vi "OriginalDigitizerLiveNew.vi"() -> ()   [LabVIEW 2020]
doc: "Example Description:\nThis example demonstrates how to enable Time Interleaved Sampling with the NI 5772 adapter module to achieve a sampling rate of 1.6GS/s. This example continuously acquires records of analog input data from the NI 5772 adapter module. It allows you to select an AI channel, trigger type, and record size. This VI must be compiled before it is run. \n\nRunning the VI:\nThis VI must be run from the NI 5772 - Getting Started (Host).vi. Refer to the host VI documentation for steps regarding running and configuring the FPGA VI. \n\nExecution Steps:\nRefer to the Block Diagram of this VI for execution comments."
uses:
  Controls/AI Trigger Type.ctl
  Controls/Aquire State.ctl
  Controls/DigitizerState.ctl
  <vilib>/Platform/TimedLoop/XDataNode/timing_clust.ctl
  <vilib>/Platform/TimedLoop/XDataNode/nitl_modes.ctl
  <vilib>/Platform/TimedLoop/XDataNode/wakeup.ctl
  Controls/NeighbouringAvgStates.ctl
  <vilib>/rvi/Emulation/niFpgaGetClockAttributes.vi
  <vilib>/rvi/Emulation/niFpgaSctlEmulationGetInTimedLoop.vi
  <vilib>/rvi/Emulation/niFpgaEmulationReportErrorSimple.vi
  <vilib>/rvi/eio/common/nirviEmuTemplateMethod_errors.vi
  <vilib>/rvi/Emulation/niFpgaCriticalErrorInLSC.vi
  <vilib>/rvi/Emulation/niFpgaEmulationIsFPGAContextNoSignature.vi
  <vilib>/rvi/errors/niFpgaSetErrorForExecOnDevCompSimple.vi
  <vilib>/rvi/eio/common/nirviEmuReportErrorAndStop.vi
  <vilib>/rvi/DataTransferAndStorage/Container/Common/niFpgaContainerGetUniqueNameForEmu.vi
  <vilib>/rvi/FIFO/Fifo_Resource/nirvififoEmulationSetSize.vi
  <vilib>/rvi/FIFO/Fifo_Resource/nirviFifoEmulationQueueMgr.vi
  <instcachedir>/0/nirviFifoEmulationQueueMgr_E5CAEC123FF24DC58D834DCA3CDAA9B5.lvgen/nirviFifoEmulationQueueMgr_E5CAEC123FF24DC58D834DCA3CDAA9B5_003.vi
  <vilib>/Utility/error.llb/Clear Errors.vi
  <vilib>/rvi/FIFO/Fifo_Resource/nirvififoEmulationCreateLock.vi
  <vilib>/rvi/Emulation/niFpgaProcessEmulError.vi
  <vilib>/rvi/FIFO/Fifo_Resource/nirvififoEmulationObtainLock.vi
  <vilib>/rvi/FIFO/Fifo_Resource/nirvififoEmulationReleaseLock.vi
  <vilib>/rvi/occurrence/nirviWaitOnOccurrenceBase.vi
  <vilib>/rvi/errors/nirviReportUnexpectedCaseInternalError.vi
  <vilib>/rvi/errors/nirviReportUnexpectedCaseInternalError (U32).vi
  <vilib>/rvi/FIFO/Fifo_Resource/nirvififoEmulationDetermineInputValidOut.vi
  <vilib>/rvi/interface/RandomDataEmulation/niFpgaRandomDataHandleErrors.vi
  <instcachedir>/0/nirviFifoEmulationQueueMgr_E5CAEC123FF24DC58D834DCA3CDAA9B5.lvgen/nirviFifoEmulationQueueMgr_E5CAEC123FF24DC58D834DCA3CDAA9B5_004.vi
  <instcachedir>/0/nirviFifoEmulationQueueMgr_E5CAEC123FF24DC58D834DCA3CDAA9B5.lvgen/nirviFifoEmulationQueueMgr_E5CAEC123FF24DC58D834DCA3CDAA9B5_000.vi
  <instrlib>/_niInstr/Basic Elements/v1/FPGA/Private/Count Up U32.vi
  <vilib>/eio/EIONode/EIONode.xnode
  <vilib>/Platform/TimedLoop/XDataNode/XDataNode.xnode
  <vilib>/rvi/DataTransferAndStorage/Container/XNode/niFpgaContainer.xnode
  <vilib>/rvi/FIFO/Fifo_Resource/nirvififoEmulationRead.vi
  <vilib>/rvi/FIFO/Fifo_Resource/nirvififoEmulationWrite.vi
  <vilib>/rvi/interface/RandomDataEmulation/nirviRandomDataFpgaReadWriteTemplate.vi
  <vilib>/Platform/TimedLoop/XDataNode/XDNodeRunTimeDep.lvlib
  <instrlib>/_niInstr/Basic Elements/v1/FPGA/niInstr Basic Elements v1 FPGA.lvlib
panel:
  out "count out":u32
  in  "Trig Width":u32
  in  "vi/nGenTrig":bool
  out "Trig In":u32
  in  "Clear TrigIn Count":bool
  out "Avg State":T1
  out "Element RemovedFIFO":u64
  out "F to H FIFO Overflow? 2":bool caption="FIFO Overflow?"
  in  "Align TimeOut":u16=50
  in  "WaitForWave\nCompletion [cycles]":u16
  out "AvgCount":u16=1
  in  "AvgCount_powerOf2":i16=1
  in  "DS":u8
  in  "Trigger":bool=TRUE
  out "Acquire State":T2
  in  "Delay Cycles":u16=512 caption="Samples Per Trigger" min=1 step=1
  out "TS FIFO In Overflow?":bool caption="FIFO Overflow?"
  in  "Samples Per Trigger":u16=512 min=1 step=1
  in  "Arm Trigger":bool
  in  "User Command Commit":bool
  in  "User Command":u8
  out "User Command Idle":bool
  out "User Command Status":u8
  in  "User Data 0":u16
  in  "User Data 1":u8
  out "PLL Locked":bool
  out "User Error":bool
  out "Configured?":bool
  out "DMA FIFO Overflow?":bool caption="FIFO Overflow?"
  in  "Trigger Level":i16
  in  "Trigger Type":T3
  # "Resource Configuration"
  # "Analog Input"
  # "Clock Configuration"
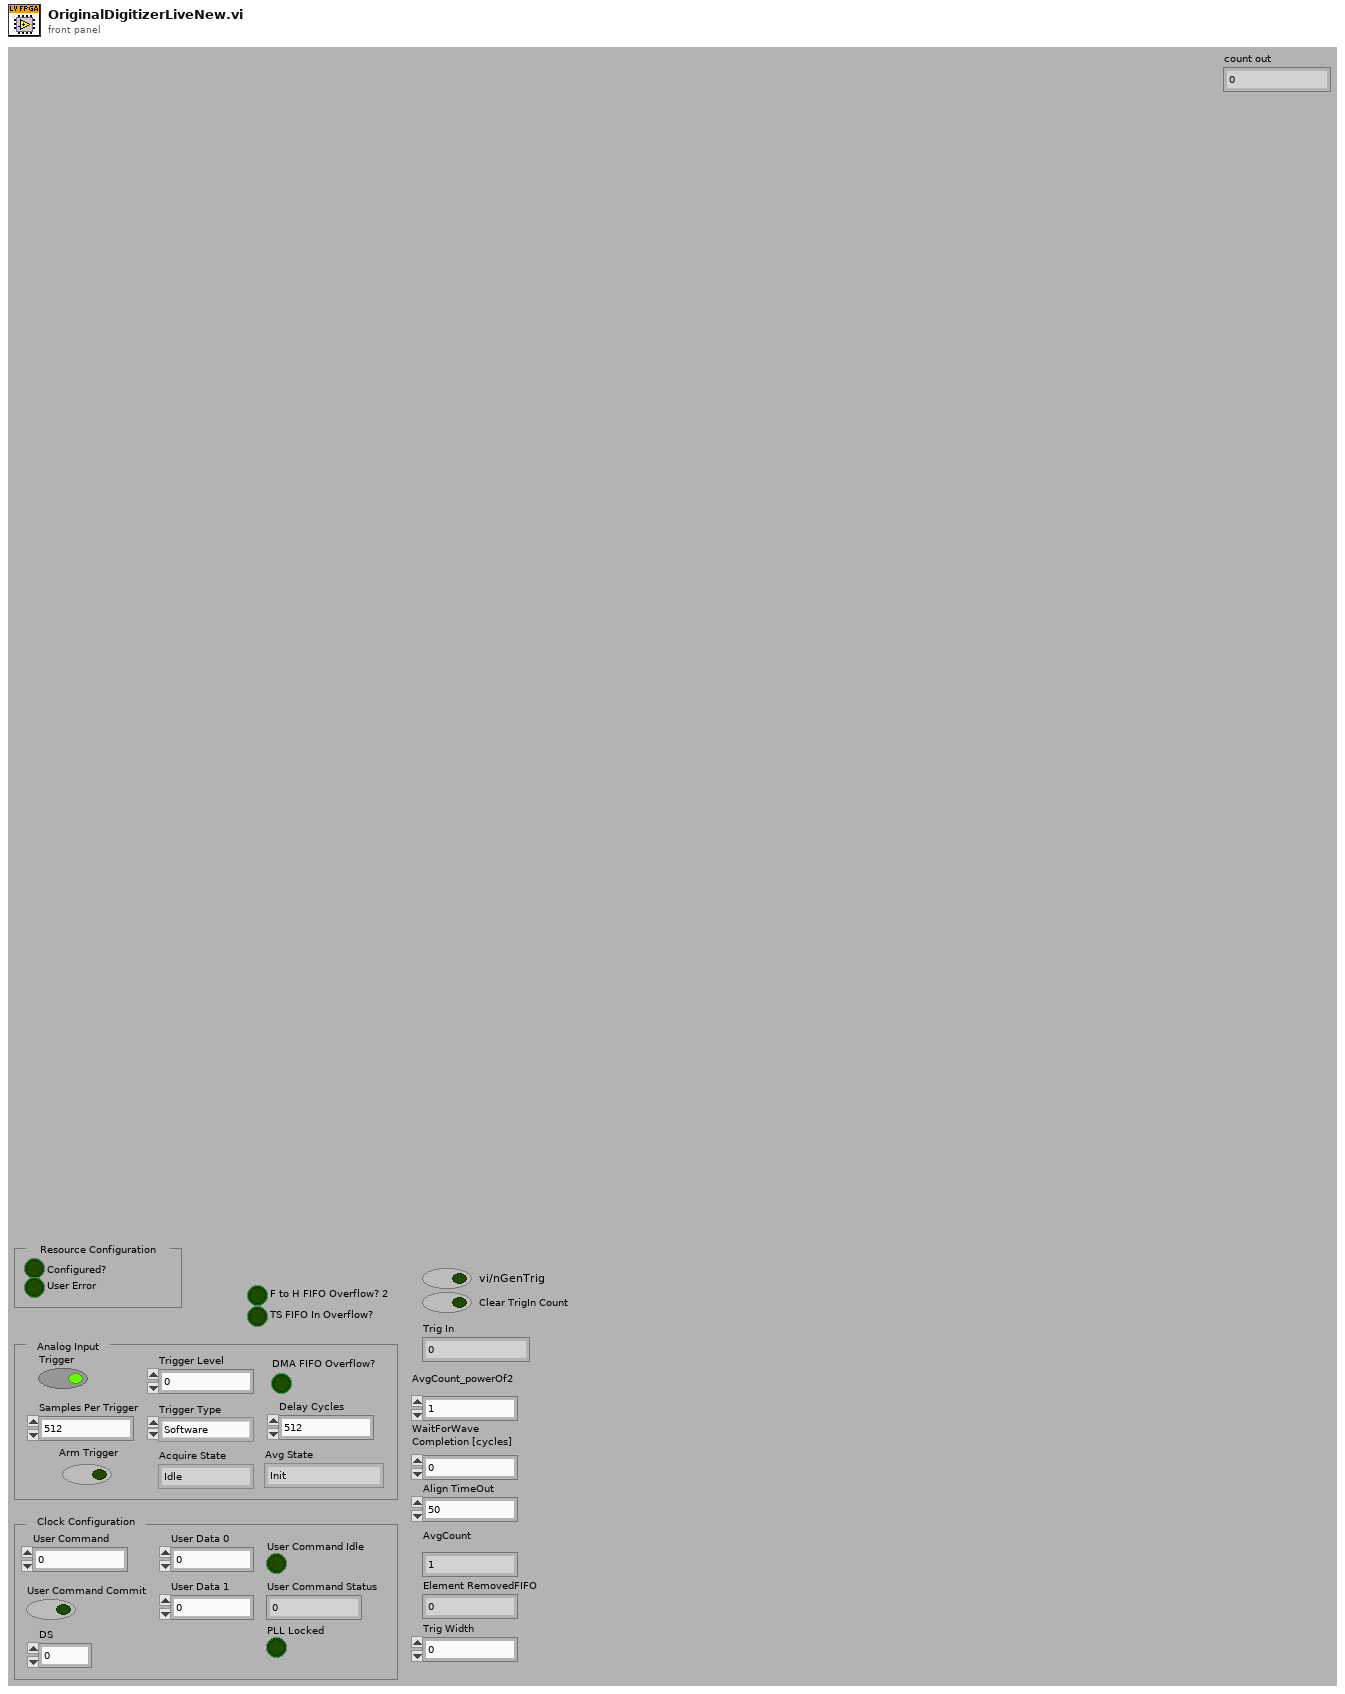
[diagram p1: front panel]
types:
  T1 = typedef "DigitizerState.ctl" = enum16{"Init", "Clear Accumulator", "Build Accumulator", "GetData", "SetData", "AverageCountCheck", "SendtoHost"}
  T2 = typedef "Aquire State.ctl" = enum8{"Idle", "Wait for Trigger", "AlignWave", "Hold Aquire", "Acquire", "WaitForWaveCompletion", "CheckAvg"}
  T3 = typedef "AI Trigger Type.ctl" = enum8{"Software", "Data Edge"}
  T4 = typedef "NeighbouringAvgStates.ctl" = enum16{"Read_noDS", "Write1_noDS", "Write2_noDS"}
  T5 = typedef "XDNodeRunTimeDep.lvlib/timing_clust.ctl" = cluster{"Expected End [f-1]":u64, "Actual End [f-1]":u64, "Finished Late? [f-1]":bool, "Expected End [i-1]":u64, "Actual End [i-1]":u64, "Finished Late? [i-1]":bool, "Expected Start [i]":u64, "Actual Start [i]":u64, "Expected Start [f]":u64, "Actual Start [f]":u64, "Source Name":string, "Structure Name":string, "Period":i64, "Deadline":i64, "Offset":i64, "Start":i64, "Priority":i32, "Timeout":i32, "Mode":T6, "Wakeup Reason":T7, "Error":errorcluster, "Source Type":string, "Secondary Source Type":string, "Global End Time":u64, "Global Start Time":u64, "Frame Duration":u64, "Iteration Duration":u64, "Assigned CPU":i32, "I/O Scan Engine Mode":u32}
  T6 = typedef "XDNodeRunTimeDep.lvlib/nitl_modes.ctl" = enum32{"No Change", "Process missed periods, maintain original phase", "Discard missed periods, maintain original phase", "Process missed periods, ignore original phase", "Discard missed periods, ignore original phase"}
  T7 = typedef "XDNodeRunTimeDep.lvlib/wakeup.ctl" = enum32{"Normal", "Aborted", "Asynchronous wakeup", "Timing source error", "Timed loop error", "Timeout"}
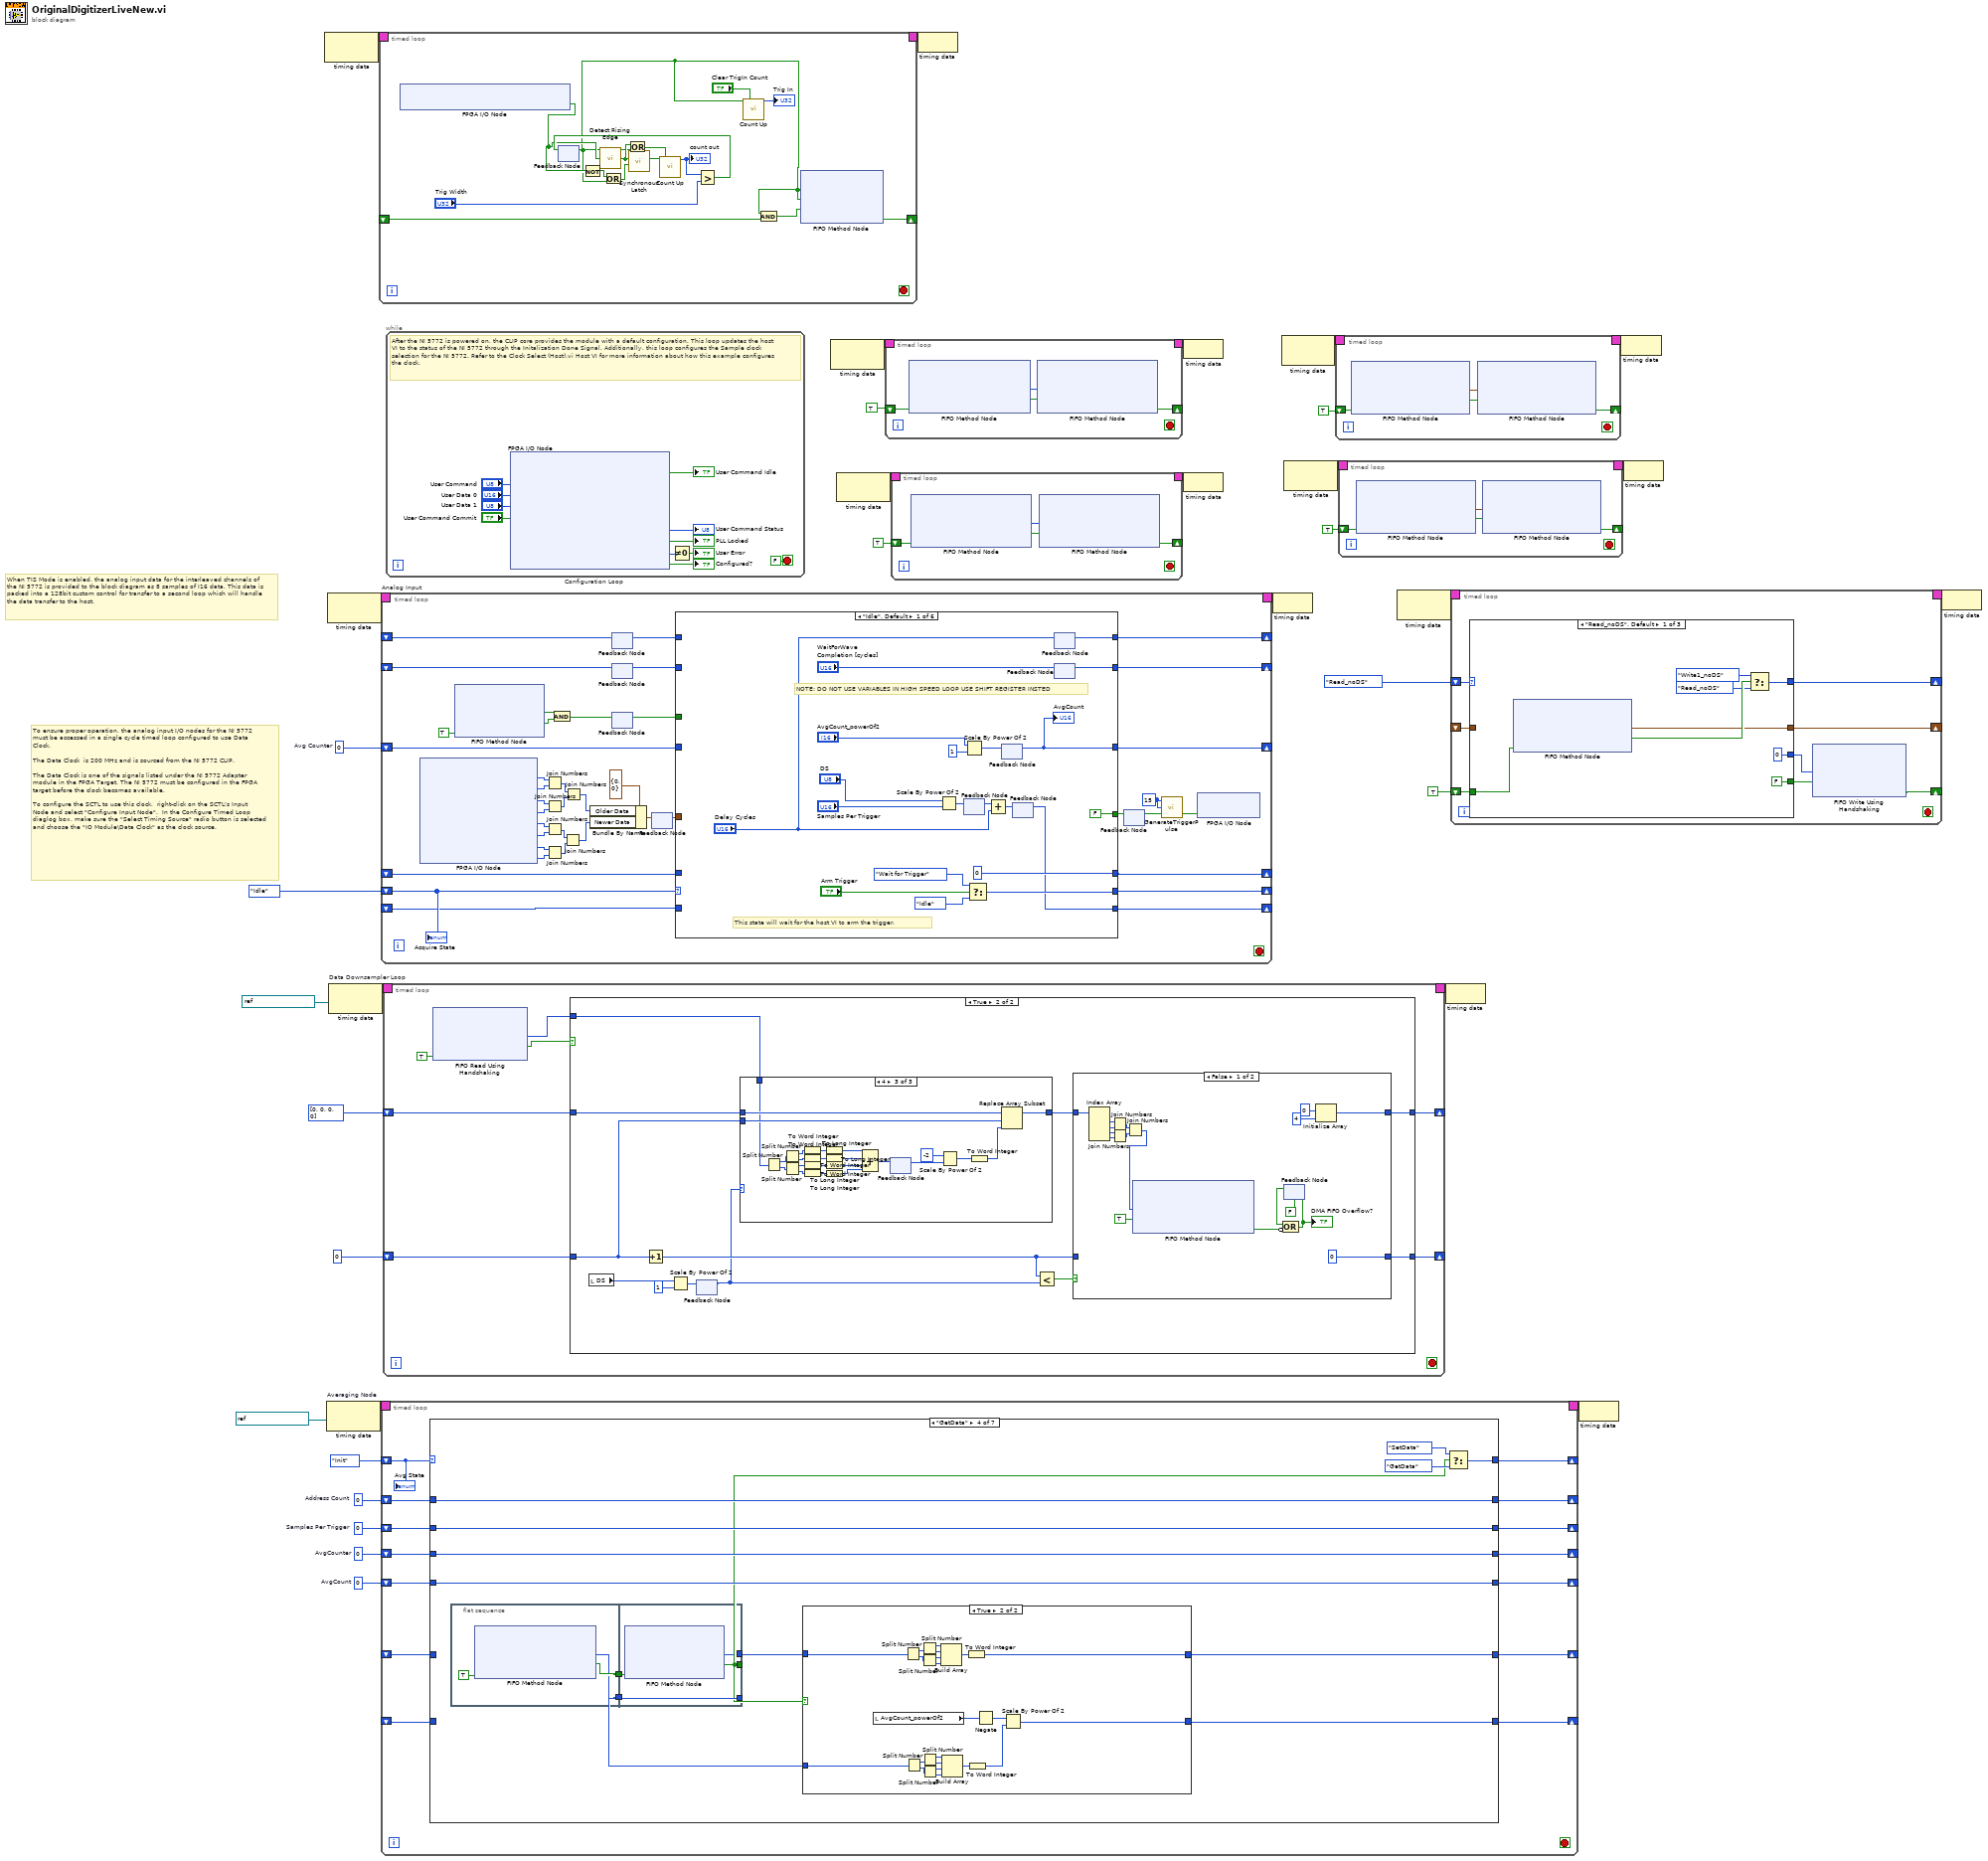
[diagram p0: block diagram]
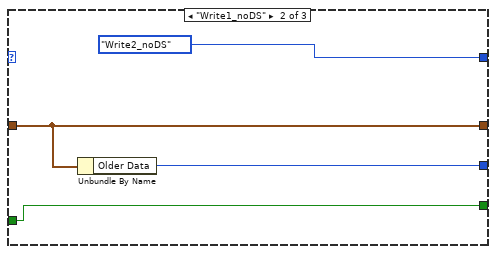
[diagram p2: hidden frame]
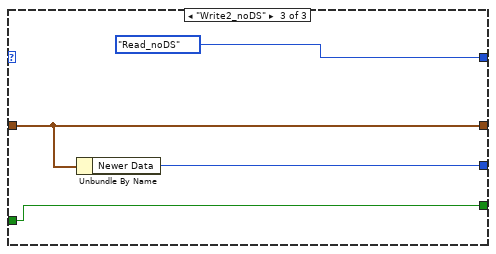
[diagram p3: hidden frame]
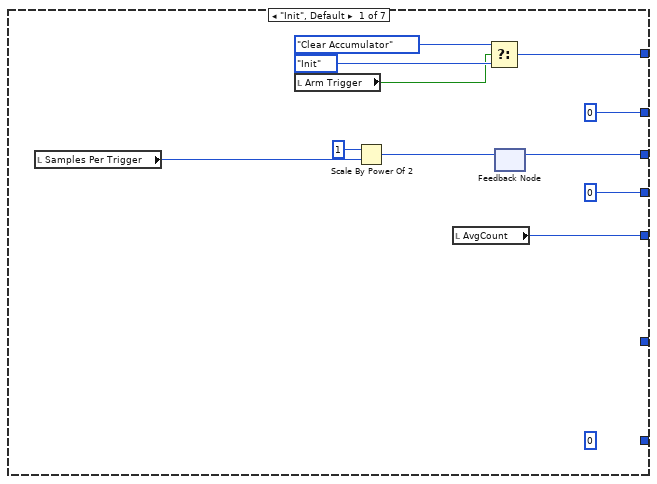
[diagram p4: hidden frame]
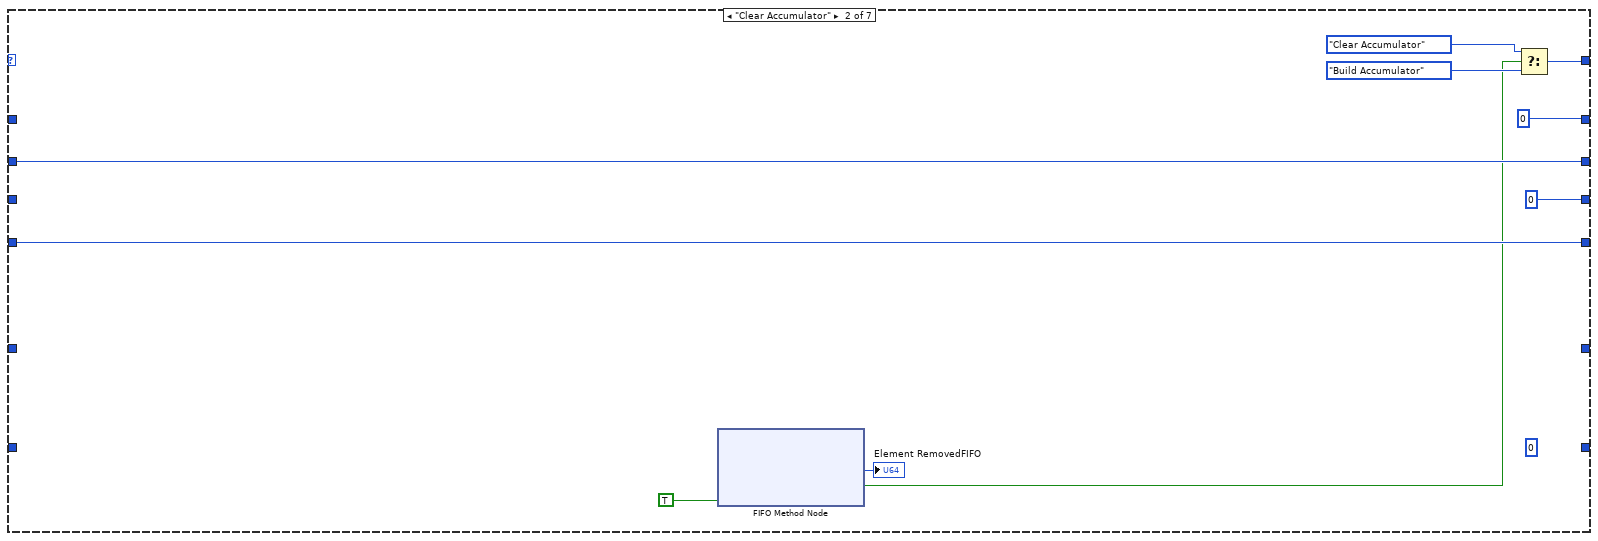
[diagram p5: hidden frame]
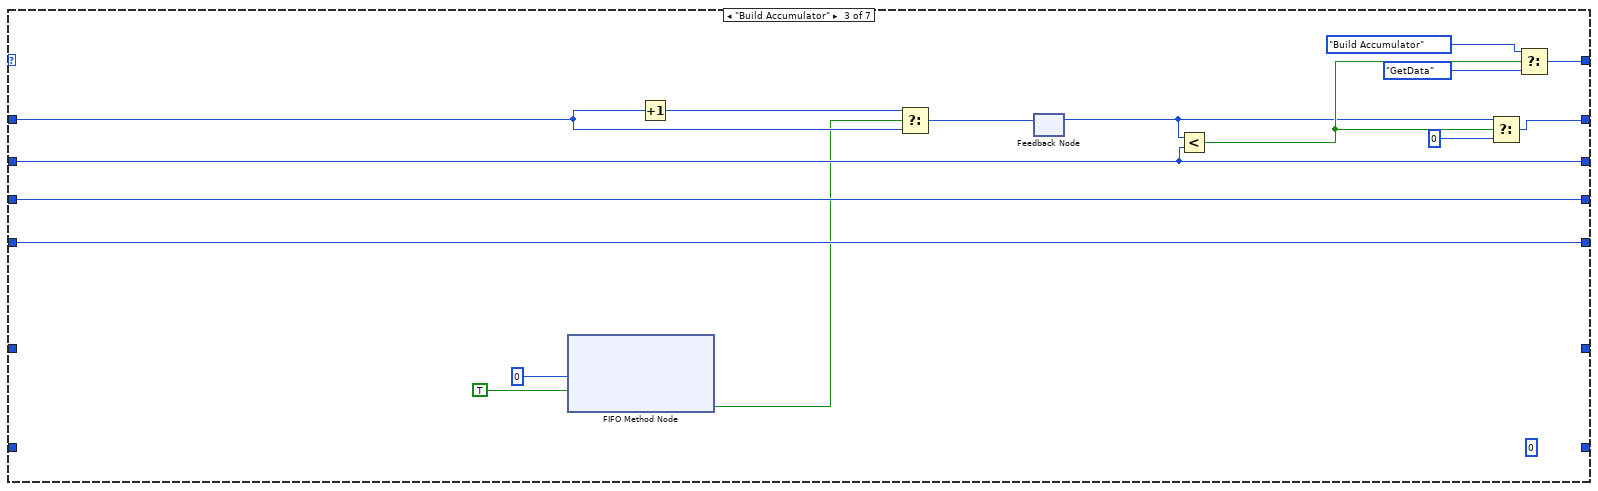
[diagram p6: hidden frame]
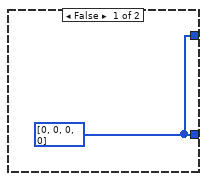
[diagram p7: hidden frame]
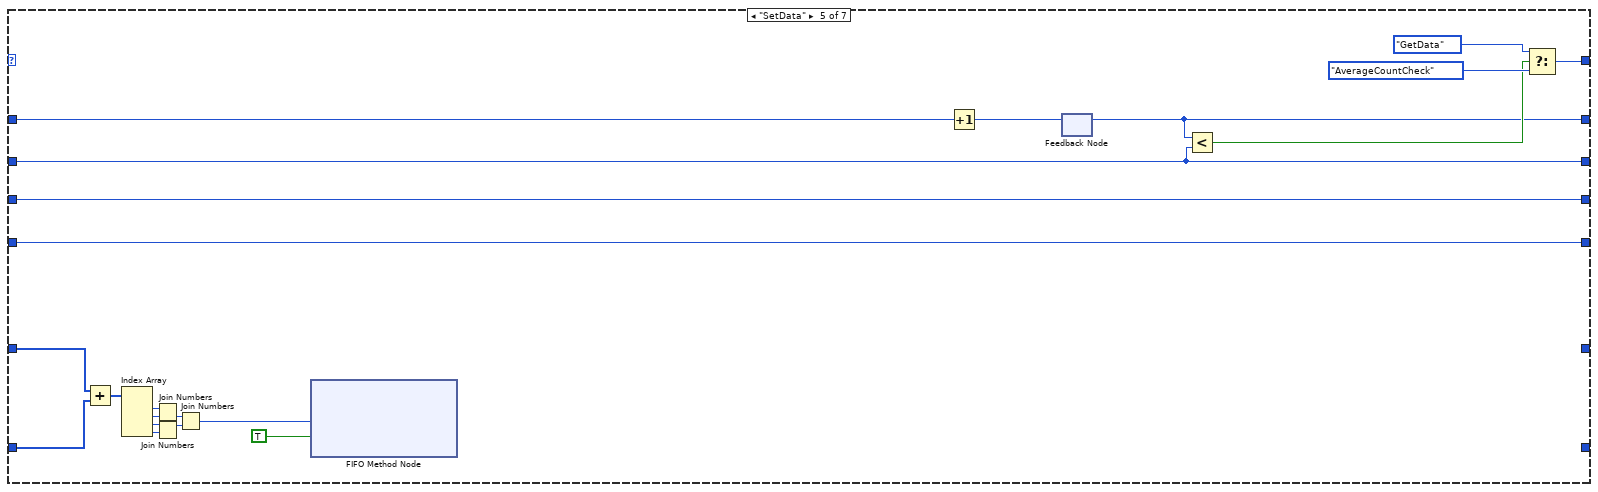
[diagram p8: hidden frame]
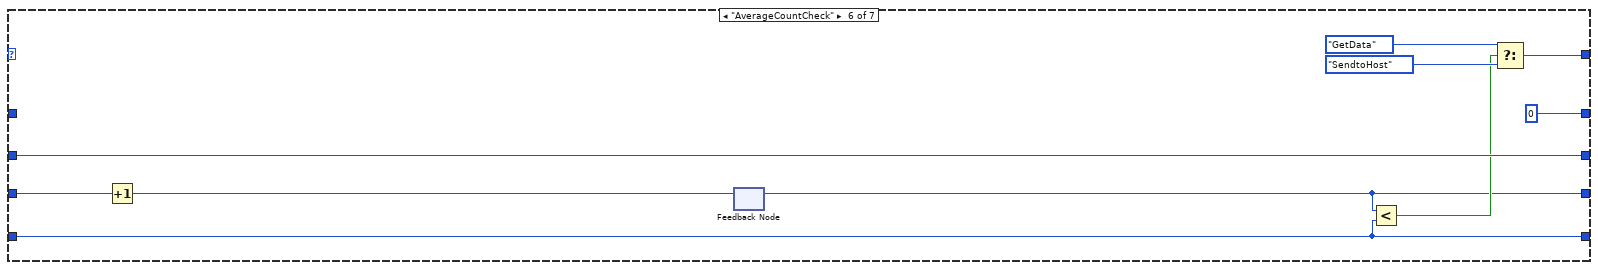
[diagram p9: hidden frame]
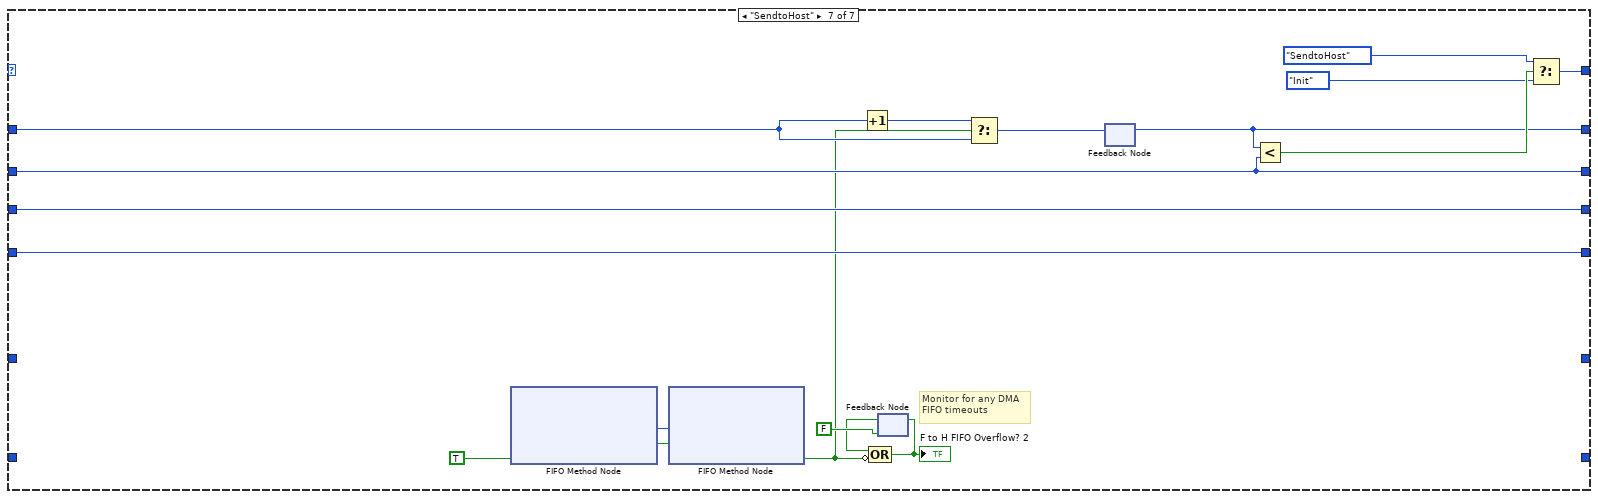
[diagram p10: hidden frame]
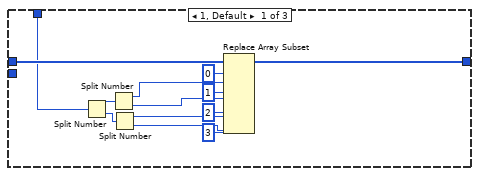
[diagram p13: hidden frame]
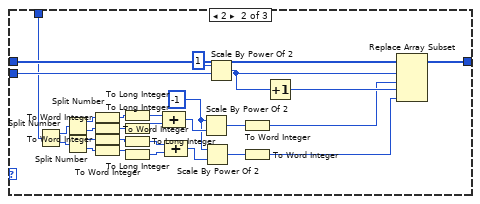
[diagram p14: hidden frame]
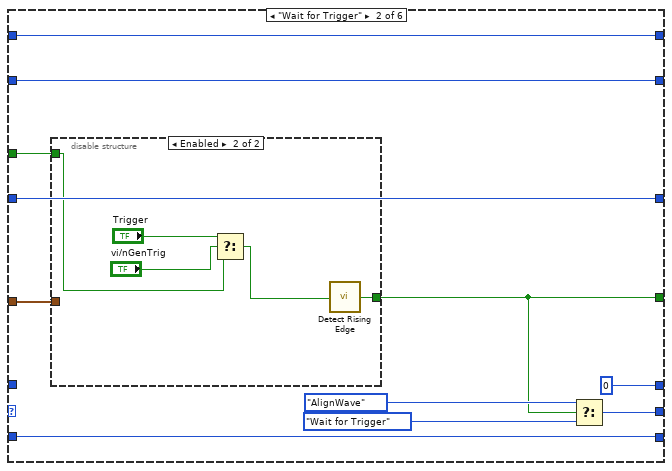
[diagram p15: hidden frame]
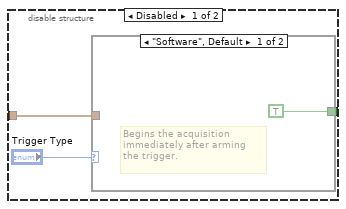
[diagram p16: hidden frame]
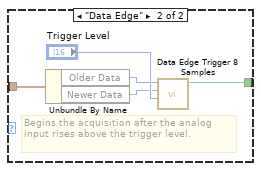
[diagram p17: hidden frame]
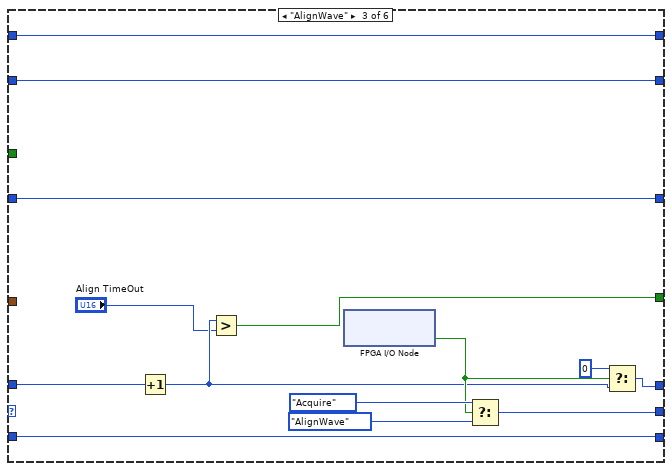
[diagram p18: hidden frame]
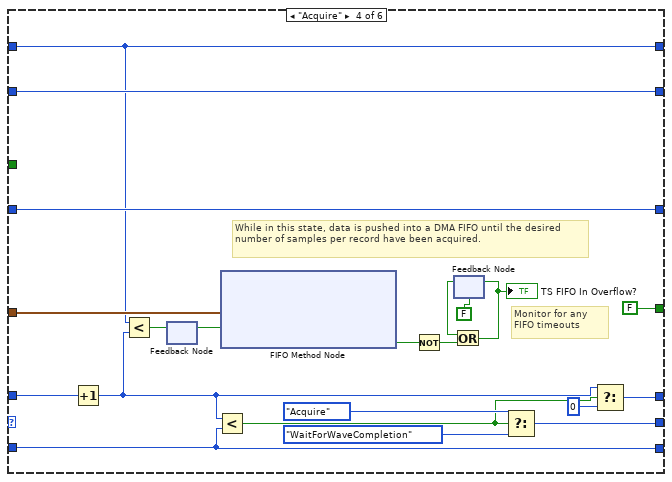
[diagram p19: hidden frame]
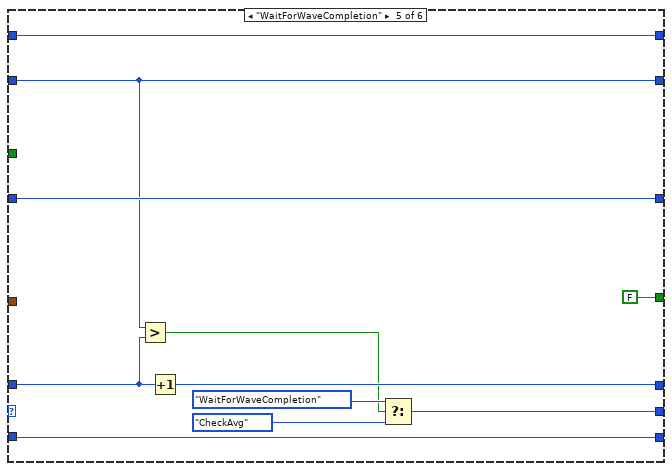
[diagram p20: hidden frame]
diagram:
  w11 = u16 0  # AvgCounter
  w13 = u32 0  # Address Count
  w12 = u16 0  # AvgCount
  w14 = u16 0  # Samples Per Trigger
  w27 = u16 0  # Avg Counter
  # "When TIS Mode is enabled, the analog input data for the interleaved channels of the NI 5772 is provided to the block diagram as 8 samples of I16 data. This data is packed into a 128bit custom control for transfer to a second loop which will handle the data transfer to the host."
  # "To ensure proper operation, the analog input I/O nodes for the NI 5772 must be accessed in a single cycle timed loop configured to use Data Clock. \n\nThe Data Clock  is 200 MHz and is sourced from the NI 5772 CLIP.\n\nThe Data Clock is one of the signals listed under the NI 5772 Adapter module in the FPGA Target. The NI 5772 must be configured in the FPGA target before the clock becomes available. \n\nTo configure the SCTL to use this clock,  right-click on the SCTL's Input Node and select \"Configure Input Node\".  In the Configure Timed Loop diaglog box, make sure the \"Select Timing Source\" radio button is selected and choose the \"IO Module\\Data Clock\" as the clock source."
  n1 = node-c288() -> (w10:T5)  [unwired: 1 in]
  n2 = node-c288 "Averaging Node"(refnum<k21> "100 MHz Clock" ("Source Name")) -> (w18:T5)
  n3 = node-c288() -> (w35:T5)  [unwired: 1 in]
  n4 = node-c288(refnum<k21> "200 MHz Clock" ("Source Name")) -> (w32:T5)
  n5 = timed-loop {
    timing: w10 -> [_]
    timing-out: [_] -> w9
    shift-right: [w50] -> _
    shift-left: _ -> [w49]
    stop <- _ stop-if-true
    n6 = xnode "FPGA I/O Node"() -> ("IO Module\\Asynchronous Trigger Input"=w38:bool)  [unwired: 1 in, 1 out]
    n7 = feedback #1() -> (w36:bool)  [unwired: 1 in]
    n8 = Not(x=w38) -> (.not. x?=w42:bool)
    n9 = call <instrlib>:"Detect Rising Edge.vi"("signal"=w38) -> ("edge detected"=w40:bool)  [unwired: 14 in]
    n10 = Or(x=w42, y=w36) -> (x .or. y?=w43:bool)
    n11 = Or(x=w40, y=w36) -> (x .or. y?=w41:bool)
    n12 = call <instrlib>:"Synchronous Latch.vi"("clear"=w43, "set"=w40) -> ("out"=w45:bool)  [unwired: 9 in]
    n13 = call-poly <instrlib>:"Count Up.vi"("increment"=w45, "reset"=w41) -> ("count out"=w46:u32)  [unwired: 13 in]
    "count out" <- w46
    n14 = Greater?(x=w46, y="Trig Width") -> (0:w44:bool)
    n15 = feedback-in #1(w44) -> ()
    n16 = call-poly <instrlib>:"Count Up.vi"("increment"=w36, "reset"="Clear TrigIn Count") -> ("count out"=→"Trig In":u32)  [unwired: 13 in]
    n17 = And(x=w36, y=w49) -> (x .and. y?=w37:bool)
    n18 = xnode ("FIFO Method Node")("Element"=w36, "Input Valid"=w37) -> ("Ready for Input"=w50:bool)  [unwired: 1 in, 1 out]
  }
  n19 = timed-loop {
    timing: w18 -> [_]
    timing-out: [_] -> w17
    shift-right: [w61] -> _
    shift-left: DigitizerState."Init" -> [w66]
    shift-right: [w60] -> _
    shift-left: w14 -> [w65]
    shift-right: [w57] -> _
    shift-left: w11 -> [w62]
    shift-right: [w58] -> _
    shift-left: w12 -> [w63]
    shift-right: [w59] -> _
    shift-left: w13 -> [w64]
    shift-right: [w53] -> _
    shift-left: _ -> [w56]
    shift-right: [w55] -> _
    shift-left: _ -> [w54]
    stop <- _ stop-if-true
    n20 = case shown="\"GetData\"" w66 {
      tunnel: w65 -> [_ w83 w95 w116 w159 w177 w186]
      tunnel: w64 -> [_ _ w90 w117 w167 _ w180]
      tunnel: w63 -> [_ w87 w103 w115 w166 w171 w194]
      tunnel: w62 -> [_ _ w102 w114 w165 w176 w195]
      tunnel: [w71 w86 w101 w112 w158 w173 w183] -> w61
      tunnel: [w67 w83 w95 w116 w159 w177 w186] -> w60
      tunnel: [u32 0 ("Address Count") u32 0 ("Address Count") w94 w117 w147 u32 0 ("f") w178] -> w59
      tunnel: [w72 w87 w103 w115 w166 w171 w194] -> w58
      tunnel: [u16 0 ("AvgCounter") u16 0 ("AvgCounter") w102 w114 w165 w168 w195] -> w57
      tunnel: w56 -> [_ _ _ _ w149 _ _]
      tunnel: [_ _ _ w109 _ _ _] -> w55
      tunnel: w54 -> [_ _ _ _ w150 _ _]
      tunnel: [_ _ _ w108 _ _ _] -> w53
      frame "Init", Default {
        (unwired) u64 0
        n21 = local read "Samples Per Trigger"() -> (w69:u16)
        n22 = local read "Arm Trigger"() -> (w73:bool)
        n23 = Scale By Power Of 2(n=i16 1, x=w69) -> (x*2^n=w70:u16)
        n24 = local read "AvgCount"() -> (w72:u16)
        n25 = Select(t=DigitizerState."Clear Accumulator", s=w73, f=DigitizerState."Init") -> (s? t:f=w71:T1)
        n26 = feedback-in #2(w70) -> ()
        n27 = feedback #2() -> (w67:u16)  [unwired: 1 in]
      }
      frame "Clear Accumulator" {
        (unwired) u64 0
        n28 = xnode ("FIFO Method Node")("Ready for Output"=TRUE) -> ("Element"=→"Element RemovedFIFO":u64, "Output Valid"=w78:bool)  [unwired: 1 in, 1 out]
        n29 = Select(t=DigitizerState."Clear Accumulator", s=w78, f=DigitizerState."Build Accumulator") -> (s? t:f=w86:T1)
      }
      frame "Build Accumulator" {
        (unwired) u64 0
        n30 = xnode ("FIFO Method Node")("Element"=u64 0, "Input Valid"=TRUE) -> ("Ready for Input"=w89:bool)  [unwired: 1 in, 1 out]
        n31 = Increment(x=w90) -> (x+1=w96:u32)
        n32 = Select(t=w96, s=w89, f=w90) -> (s? t:f=w91:u32)
        n33 = feedback-in #3(w91) -> ()
        n34 = feedback #3() -> (w88:u32)  [unwired: 1 in]
        n35 = Less?(x=w88, y=w95) -> (x < y?=w92:bool)
        n36 = Select(t=w88, s=w92, f=u32 0) -> (s? t:f=w94:u32)
        n37 = Select(t=DigitizerState."Build Accumulator", s=w92, f=DigitizerState."GetData") -> (s? t:f=w101:T1)
      }
      frame "GetData" {
        n38 = flat-sequence {
          tunnel: [w119] -> w107
          tunnel: [w118] -> w106
          tunnel: [w124] -> w113
          tunnel: w107 -> [w121]
          tunnel: w106 -> [w124]
          tunnel: [w123] -> w105
          tunnel: [w122] -> w104
          frame #0 {
            n39 = xnode ("FIFO Method Node")("Ready for Output"=TRUE) -> ("Element"=w118:u64, "Output Valid"=w119:bool)  [unwired: 1 in, 1 out]
          }
          frame #1 {
            n40 = xnode ("FIFO Method Node")("Ready for Output"=w121) -> ("Element"=w123:u64, "Output Valid"=w122:bool)  [unwired: 1 in, 1 out]
          }
        }
        n41 = case shown="True" w104 {
          tunnel: w113 -> [_ w128]
          tunnel: w105 -> [_ w129]
          tunnel: [w125 w127] -> w108
          tunnel: [w125 w126] -> w109
          frame False {
            w125 = i16[] [0, 0, 0, 0]
          }
          frame True {
            n42 = local read "AvgCount_powerOf2"() -> (w131:i16)
            n43 = Split Number(x=w129) -> (hi(x)=w132:u32, lo(x)=w133:u32)
            n44 = Split Number(x=w128) -> (hi(x)=w145:u32, lo(x)=w144:u32)
            n45 = Split Number(x=w132) -> (hi(x)=w134:u16, lo(x)=w135:u16)
            n46 = Split Number(x=w133) -> (hi(x)=w136:u16, lo(x)=w137:u16)
            n47 = Split Number(x=w145) -> (hi(x)=w143:u16, lo(x)=w142:u16)
            n48 = Split Number(x=w144) -> (hi(x)=w141:u16, lo(x)=w140:u16)
            n49 = Build Array(w134, w135, w136, w137) -> (w138:u16[])
            n50 = Build Array(w143, w142, w141, w140) -> (w139:u16[])
            n51 = To Word Integer(number=w138) -> (16bit integer=w126:i16[])
            n52 = To Word Integer(number=w139) -> (16bit integer=w146:i16[])
            n53 = Negate(x=w131) -> (-x=w130:i16)
            n54 = Scale By Power Of 2(n=w130, x=w146) -> (x*2^n=w127:i16[])
          }
        }
        n55 = Select(t=DigitizerState."SetData", s=w104, f=DigitizerState."GetData") -> (s? t:f=w112:T1)
      }
      frame "SetData" {
        n56 = Add(x=w150, y=w149) -> (x+y=w157:i16[])
        n57 = Index Array(array=w157) -> (element #1=w154:i16, element #2=w153:i16, element #3=w152:i16, element #4=w151:i16)  [unwired: 4 in]
        n58 = Join Numbers(hi=w154, lo=w153) -> ((hi.lo)=w156:u32)
        n59 = Join Numbers(hi=w152, lo=w151) -> ((hi.lo)=w155:u32)
        n60 = Join Numbers(hi=w156, lo=w155) -> ((hi.lo)=w148:u64)
        n61 = xnode ("FIFO Method Node")("Element"=w148, "Input Valid"=TRUE) -> ()  [unwired: 1 in, 2 out]
        n62 = Increment(x=w167) -> (x+1=w160:u32)
        n63 = feedback-in #4(w160) -> ()
        n64 = feedback #4() -> (w147:u32)  [unwired: 1 in]
        n65 = Less?(x=w147, y=w159) -> (x < y?=w161:bool)
        n66 = Select(t=DigitizerState."GetData", s=w161, f=DigitizerState."AverageCountCheck") -> (s? t:f=w158:T1)
      }
      frame "AverageCountCheck" {
        n67 = Increment(x=w176) -> (x+1=w172:u16)
        n68 = feedback-in #5(w172) -> ()
        n69 = feedback #5() -> (w168:u16)  [unwired: 1 in]
        n70 = Less?(x=w168, y=w171) -> (x < y?=w170:bool)
        n71 = Select(t=DigitizerState."GetData", s=w170, f=DigitizerState."SendtoHost") -> (s? t:f=w173:T1)
      }
      frame "SendtoHost" {
        # "Monitor for any DMA FIFO timeouts"
        n72 = xnode ("FIFO Method Node")("Ready for Output"=TRUE) -> ("Element"=w189:u64, "Output Valid"=w190:bool)  [unwired: 1 in, 1 out]
        n73 = xnode ("FIFO Method Node")("Element"=w189, "Input Valid"=w190) -> ("Ready for Input"=w179:bool)  [unwired: 1 in, 1 out]
        n74 = Increment(x=w180) -> (x+1=w187:u32)
        n75 = feedback #6(FALSE) -> (w192:bool)
        n76 = Compound Arithmetic op=OR(w192, invert w179) -> (w191:bool)
        "F to H FIFO Overflow? 2" <- w191
        n77 = feedback-in #6(w191) -> ()
        n78 = Select(t=w187, s=w179, f=w180) -> (s? t:f=w181:u32)
        n79 = feedback-in #7(w181) -> ()
        n80 = feedback #7() -> (w178:u32)  [unwired: 1 in]
        n81 = Less?(x=w178, y=w186) -> (x < y?=w185:bool)
        n82 = Select(t=DigitizerState."SendtoHost", s=w185, f=DigitizerState."Init") -> (s? t:f=w183:T1)
      }
    }
    "Avg State" <- w66
  }
  n83 = timed-loop "Analog Input" {
    timing: w35 -> [_]
    timing-out: [_] -> w34
    shift-right: [w236] -> _
    shift-left: Aquire_State."Idle" ("Acquire State") -> [w226]
    shift-right: [w237] -> _
    shift-left: _ -> [w227]
    shift-right: [w235] -> _
    shift-left: _ -> [w225]
    shift-right: [w210] -> _
    shift-left: w27 -> [w211]
    shift-right: [w203] -> _
    shift-left: _ -> [w202]
    shift-right: [w201] -> _
    shift-left: _ -> [w200]
    stop <- _ stop-if-true
    w213 = u16 15 ("Pulse Width On [cycles]")
    n84 = xnode "FPGA I/O Node"() -> ("IO Module\\AI 1 Data N-3"=w218:i16, "IO Module\\AI 0 Data N-3"=w217:i16, "IO Module\\AI 1 Data N-2"=w216:i16, "IO Module\\AI 0 Data N-2"=w215:i16, "IO Module\\AI 1 Data N-1"=w219:i16, "IO Module\\AI 0 Data N-1"=w220:i16, "IO Module\\AI 1 Data N"=w221:i16, "IO Module\\AI 0 Data N"=w222:i16)  [unwired: 8 in, 8 out]
    n85 = xnode ("FIFO Method Node")("Ready for Output"=TRUE) -> ("Element"=w206:bool, "Output Valid"=w207:bool)  [unwired: 1 in, 1 out]
    n86 = Join Numbers(hi=w218, lo=w217) -> ((hi.lo)=w230:u32)
    n87 = Join Numbers(hi=w216, lo=w215) -> ((hi.lo)=w232:u32)
    n88 = Join Numbers(hi=w219, lo=w220) -> ((hi.lo)=w231:u32)
    n89 = Join Numbers(hi=w221, lo=w222) -> ((hi.lo)=w233:u32)
    n90 = And(x=w206, y=w207) -> (x .and. y?=w205:bool)
    n91 = Join Numbers(hi=w231, lo=w233) -> ((hi.lo)=w223:u64)
    n92 = Join Numbers(hi=w230, lo=w232) -> ((hi.lo)=w224:u64)
    n93 = Bundle By Name(cluster=cluster{"Older Data":u64, "Newer Data":u64} {"Older Data"=0, "Newer Data"=0} ("Element"), "Older Data"=w224, "Newer Data"=w223) -> (w228:cluster{"Older Data":u64, "Newer Data":u64})
    n94 = feedback-in #8(w200) -> ()
    n95 = feedback #8() -> (w199:u16)  [unwired: 1 in]
    n96 = feedback-in #9(w202) -> ()
    n97 = feedback #9() -> (w198:u16)  [unwired: 1 in]
    n98 = feedback-in #10(w205) -> ()
    n99 = feedback #10() -> (w204:bool)  [unwired: 1 in]
    n100 = feedback #11() -> (w234:cluster{"Older Data":u64, "Newer Data":u64})  [unwired: 1 in]
    n101 = feedback-in #11(w228) -> ()
    n102 = case shown="\"Idle\", Default" w226 {
      tunnel: [u16 0 u16 0 w291 w304 w327 u16 0 ("f")] -> w237
      tunnel: w227 -> [_ _ w290 w317 w326 _]
      tunnel: [w254 w264 w294 w316 w323 w333] -> w236
      tunnel: [w252 w268 w293 w313 w328 w337] -> w235
      tunnel: w225 -> [_ w268 w293 w313 w328 w337]
      tunnel: w234 -> [_ w267 _ w312 _ _]
      tunnel: [FALSE ("edge detected") w262 w285 FALSE ("edge detected") FALSE ("edge detected") w332] -> w212
      tunnel: w211 -> [_ w261 w292 w300 w321 w338]
      tunnel: [w238 w261 w292 w300 w321 w335] -> w210
      tunnel: w204 -> [_ w260 _ _ _ _]
      tunnel: [w245 w259 w284 w298 w319 w330] -> w203
      tunnel: w198 -> [_ w259 w284 w298 w319 w330]
      tunnel: [w243 w258 w283 w297 w318 w329] -> w201
      tunnel: w199 -> [_ w258 w283 w297 w318 w329]
      frame "Idle", Default {
        # "NOTE: DO NOT USE VARIABLES IN HIGH SPEED LOOP USE SHIFT REGISTER INSTED"
        # "This state will wait for the host VI to arm the trigger."
        n103 = Scale By Power Of 2(n="DS", x="Samples Per Trigger") -> (x*2^n=w250:u16)
        n104 = feedback-in #12(w250) -> ()
        n105 = feedback #12() -> (w248:u16)  [unwired: 1 in]
        n106 = Scale By Power Of 2(n="AvgCount_powerOf2", x=u16 1) -> (x*2^n=w240:u16)
        n107 = Select(t=Aquire_State."Wait for Trigger" ("Acquire State"), s="Arm Trigger", f=Aquire_State."Idle" ("Acquire State")) -> (s? t:f=w254:T2)
        n108 = Add(x=w248, y="Delay Cycles") -> (x+y=w253:u16)
        n109 = feedback-in #13(w240) -> ()
        n110 = feedback #13() -> (w238:u16)  [unwired: 1 in]
        "AvgCount" <- w238
        n111 = feedback-in #14(w253) -> ()
        n112 = feedback #14() -> (w252:u16)  [unwired: 1 in]
        n113 = feedback-in #15("Delay Cycles") -> ()
        n114 = feedback #15() -> (w243:u16)  [unwired: 1 in]
        n115 = feedback-in #16("WaitForWave\nCompletion [cycles]") -> ()
        n116 = feedback #16() -> (w245:u16)  [unwired: 1 in]
      }
      frame "Wait for Trigger" {
        n117 = disable-structure shown="Enabled" {
          disable-tunnel: w267 -> [w270 _]
          disable-tunnel: [w269 w281] -> w262
          disable-tunnel: w260 -> [_ w278]
          frame Disabled {
            n118 = case shown="\"Software\", Default" "Trigger Type" {
              tunnel: w270 -> [_ w277]
              tunnel: [TRUE ("Trigger") w276] -> w269
              frame "Software", Default {
                # "Begins the acquisition immediately after arming the trigger."
              }
              frame "Data Edge" {
                # "Begins the acquisition after the analog input rises above the trigger level."
                n119 = Unbundle By Name(w277) -> ("Older Data"=w275:u64, "Newer Data"=w273:u64)
                n120 = call "Data Edge Trigger 8 Samples.vi"("Trigger Level"="Trigger Level", "Newer Data In"=w273, "Older Data In"=w275) -> ("Trigger"=w276:bool)  [unwired: 8 in]
              }
            }
          }
          frame Enabled {
            n121 = Select(t="Trigger", s="vi/nGenTrig", f=w278) -> (s? t:f=w280:bool)
            n122 = call <instrlib>:"Detect Rising Edge.vi"("signal"=w280) -> ("edge detected"=w281:bool)  [unwired: 14 in]
          }
        }
        n123 = Select(t=Aquire_State."AlignWave" ("Acquire State"), s=w262, f=Aquire_State."Wait for Trigger") -> (s? t:f=w264:T2)
      }
      frame "AlignWave" {
        n124 = Increment(x=w290) -> (x+1=w287:u16)
        n125 = Greater?(x=w287, y="Align TimeOut") -> (0:w285:bool)
        n126 = xnode "FPGA I/O Node"() -> ("PXI_Trig0"=w289:bool)  [unwired: 1 in, 1 out]
        n127 = Select(t=Aquire_State."Acquire" ("Acquire State"), s=w289, f=Aquire_State."AlignWave") -> (s? t:f=w294:T2)
        n128 = Select(t=u16 0, s=w289, f=w287) -> (s? t:f=w291:u16)
      }
      frame "Acquire" {
        # "Monitor for any  FIFO timeouts"
        # "While in this state, data is pushed into a DMA FIFO until the desired number of samples per record have been acquired."
        n129 = Increment(x=w317) -> (x+1=w303:u16)
        n130 = Less?(x=w297, y=w303) -> (x < y?=w308:bool)
        n131 = feedback-in #17(w308) -> ()
        n132 = feedback #17() -> (w305:bool)  [unwired: 1 in]
        n133 = Less?(x=w303, y=w313) -> (x < y?=w302:bool)
        n134 = xnode ("FIFO Method Node")("Element"=w312, "Input Valid"=w305) -> ("Ready for Input"=w307:bool)  [unwired: 1 in, 1 out]
        n135 = Not(x=w307) -> (.not. x?=w306:bool)
        n136 = feedback #18(FALSE) -> (w309:bool)
        n137 = Or(x=w309, y=w306) -> (x .or. y?=w310:bool)
        "TS FIFO In Overflow?" <- w310
        n138 = feedback-in #18(w310) -> ()
        n139 = Select(t=Aquire_State."Acquire" ("Acquire State"), s=w302, f=Aquire_State."WaitForWaveCompletion" ("Acquire State")) -> (s? t:f=w316:T2)
        n140 = Select(t=w303, s=w302, f=u16 0) -> (s? t:f=w304:u16)
      }
      frame "WaitForWaveCompletion" {
        n141 = Greater?(x=w319, y=w326) -> (0:w322:bool)
        n142 = Increment(x=w326) -> (x+1=w327:u16)
        n143 = Select(t=Aquire_State."WaitForWaveCompletion" ("Acquire State"), s=w322, f=Aquire_State."CheckAvg" ("Acquire State")) -> (s? t:f=w323:T2)
      }
      frame "CheckAvg" {
        n144 = Decrement(x=w338) -> (x-1=w335:u16)
        n145 = Not Equal To 0?(x=w335) -> (x != 0?=w332:bool)
        n146 = Select(t=Aquire_State."AlignWave" ("Acquire State"), s=w332, f=Aquire_State."Idle") -> (s? t:f=w333:T2)
      }
    }
    n147 = feedback-in #19(w212) -> ()
    n148 = feedback #19() -> (w209:bool)  [unwired: 1 in]
    n149 = call "GenerateTriggerPulse.vi"("Trigger"=w209, "Pulse Width Off [cycles]"=w213, "Pulse Width On [cycles]"=w213) -> ("Out"=w214:bool)  [unwired: 2 out]
    n150 = xnode "FPGA I/O Node"("PXI_Trig1"=w214) -> ()  [unwired: 1 in, 1 out]
    "Acquire State" <- w226
  }
  n151 = timed-loop "Data Downsampler Loop" {
    timing: w32 -> [_]
    timing-out: [_] -> w31
    shift-right: [w345] -> _
    shift-left: u16 0 -> [w347]
    shift-right: [w344] -> _
    shift-left: i16[] [0, 0, 0, 0] -> [w346]
    stop <- _ stop-if-true
    n152 = xnode ("FIFO Read Using Handshaking")("Ready for Output"=TRUE) -> ("Element"=w343:u64, "Output Valid"=w342:bool)  [unwired: 1 in, 1 out]
    n153 = case shown="True" w342 {
      tunnel: w343 -> [_ w358]
      tunnel: w347 -> [w349 w357]
      tunnel: [w349 w350] -> w345
      tunnel: w346 -> [w348 w356]
      tunnel: [w348 w351] -> w344
      frame False {
      }
      frame True {
        n154 = local read "DS"() -> (w355:u8)
        n155 = Increment(x=w357) -> (x+1=w361:u16)
        n156 = Scale By Power Of 2(n=w355, x=u8 1) -> (x*2^n=w353:u8)
        n157 = feedback #20() -> (w352:u8)  [unwired: 1 in]
        n158 = feedback-in #20(w353) -> ()
        n159 = case shown="4" w352 {
          tunnel: w356 -> [w393 w415 w438]
          tunnel: [w392 w414 w437] -> w360
          tunnel: w357 -> [_ w411 w436]
          tunnel: w358 -> [w381 w409 w431]
          frame 1, Default {
            n160 = Split Number(x=w381) -> (hi(x)=w391:u32, lo(x)=w390:u32)
            n161 = Split Number(x=w391) -> (hi(x)=w389:u16, lo(x)=w388:u16)
            n162 = Split Number(x=w390) -> (hi(x)=w387:u16, lo(x)=w386:u16)
            n163 = Replace Array Subset(array=w393, new element #1=w389, index #1=0 ("index"), new element #2=w388, index #2=1 ("index"), new element #3=w387, index #3=2 ("index"), new element #4=w386, index #4=3 ("index")) -> (w392:i16[])
          }
          frame 2 {
            w394 = i16 -1 ("n")
            n164 = Split Number(x=w409) -> (hi(x)=w421:u32, lo(x)=w420:u32)
            n165 = Split Number(x=w421) -> (hi(x)=w419:u16, lo(x)=w418:u16)
            n166 = Split Number(x=w420) -> (hi(x)=w417:u16, lo(x)=w416:u16)
            n167 = To Word Integer(number=w419) -> (16bit integer=w408:i16)
            n168 = To Word Integer(number=w418) -> (16bit integer=w406:i16)
            n169 = To Word Integer(number=w417) -> (16bit integer=w405:i16)
            n170 = To Word Integer(number=w416) -> (16bit integer=w407:i16)
            n171 = To Long Integer(number=w408) -> (32bit integer=w404:i32)
            n172 = To Long Integer(number=w406) -> (32bit integer=w403:i32)
            n173 = To Long Integer(number=w405) -> (32bit integer=w402:i32)
            n174 = To Long Integer(number=w407) -> (32bit integer=w401:i32)
            n175 = Compound Arithmetic op=unknown(w404, w403) -> (w395:i32)
            n176 = Compound Arithmetic op=unknown(w402, w401) -> (w396:i32)
            n177 = Scale By Power Of 2(n=w394, x=w395) -> (x*2^n=w397:i32)
            n178 = Scale By Power Of 2(n=w394, x=w396) -> (x*2^n=w398:i32)
            n179 = Scale By Power Of 2(n=i16 1, x=w411) -> (x*2^n=w412:u16)
            n180 = To Word Integer(number=w397) -> (16bit integer=w399:i16)
            n181 = To Word Integer(number=w398) -> (16bit integer=w400:i16)
            n182 = Increment(x=w412) -> (x+1=w413:u16)
            n183 = Replace Array Subset(array=w415, new element #1=w399, index #1=w412, new element #2=w400, index #2=w413) -> (w414:i16[])
          }
          frame 4 {
            n184 = Split Number(x=w431) -> (hi(x)=w444:u32, lo(x)=w443:u32)
            n185 = Split Number(x=w444) -> (hi(x)=w442:u16, lo(x)=w441:u16)
            n186 = Split Number(x=w443) -> (hi(x)=w440:u16, lo(x)=w439:u16)
            n187 = To Word Integer(number=w442) -> (16bit integer=w435:i16)
            n188 = To Word Integer(number=w441) -> (16bit integer=w434:i16)
            n189 = To Word Integer(number=w440) -> (16bit integer=w433:i16)
            n190 = To Word Integer(number=w439) -> (16bit integer=w432:i16)
            n191 = To Long Integer(number=w435) -> (32bit integer=w427:i32)
            n192 = To Long Integer(number=w434) -> (32bit integer=w428:i32)
            n193 = To Long Integer(number=w433) -> (32bit integer=w429:i32)
            n194 = To Long Integer(number=w432) -> (32bit integer=w430:i32)
            n195 = Compound Arithmetic op=unknown(w427, w428, w429, w430) -> (w426:i32)
            n196 = feedback-in #21(w426) -> ()
            n197 = feedback #21() -> (w422:i32)  [unwired: 1 in]
            n198 = Scale By Power Of 2(n=i16 -2, x=w422) -> (x*2^n=w424:i32)
            n199 = To Word Integer(number=w424) -> (16bit integer=w423:i16)
            n200 = Replace Array Subset(array=w438, new element=w423, index=w436) -> (w437:i16[])
          }
        }
        n201 = Less?(x=w361, y=w352) -> (x < y?=w359:bool)
        n202 = case shown="False" w359 {
          tunnel: w360 -> [w372 w380]
          tunnel: [w369 w380] -> w351
          tunnel: w361 -> [_ w379]
          tunnel: [u16 0 w379] -> w350
          frame False {
            n203 = Index Array(array=w372) -> (element #1=w376:i16, element #2=w375:i16, element #3=w374:i16, element #4=w373:i16)  [unwired: 4 in]
            n204 = Join Numbers(hi=w376, lo=w375) -> ((hi.lo)=w378:u32)
            n205 = Join Numbers(hi=w374, lo=w373) -> ((hi.lo)=w377:u32)
            n206 = Join Numbers(hi=w378, lo=w377) -> ((hi.lo)=w365:u64)
            n207 = xnode ("FIFO Method Node")("Element"=w365, "Input Valid"=TRUE) -> ("Ready for Input"=w362:bool)  [unwired: 1 in, 1 out]
            n208 = feedback #22(FALSE) -> (w366:bool)
            n209 = Compound Arithmetic op=OR(w366, invert w362) -> (w364:bool)
            "DMA FIFO Overflow?" <- w364
            n210 = feedback-in #22(w364) -> ()
            n211 = Initialize Array(i16 0 ("element"), 4 ("dimension size")) -> (w369:i16[])
          }
          frame True {
          }
        }
      }
    }
  }
  n212 = while "Configuration Loop" {
    stop <- FALSE stop-if-true
    # "After the NI 5772 is powered on, the CLIP core provides the module with a default configuration. This loop updates the host VI to the status of the NI 5772 through the Initalization Done Signal. Additionally, this loop configures the Sample clock selection for the NI 5772. Refer to the Clock Select (Host).vi Host VI for more information about how this example configures the clock."
    n213 = xnode "FPGA I/O Node"("IO Module\\User Command"="User Command", "IO Module\\User Data 0"="User Data 0", "IO Module\\User Data 1"="User Data 1", "IO Module\\User Command Commit"="User Command Commit") -> ("IO Module\\User Command Idle"=→"User Command Idle":bool, "IO Module\\User Command Status"=→"User Command Status":u8, "IO Module\\PLL Locked"=→"PLL Locked":bool, "IO Module\\User Error"=w452:u8, "IO Module\\Initialization Done"=→"Configured?":bool)  [unwired: 9 in, 9 out]
    n214 = Not Equal To 0?(x=w452) -> (x != 0?=→"User Error":bool)
  }
  n215 = node-c288() -> (w24:T5)  [unwired: 1 in]
  n216 = node-c288() -> (w22:T5)  [unwired: 1 in]
  n217 = timed-loop {
    timing: w24 -> [_]
    timing-out: [_] -> w23
    shift-right: [w459] -> _
    shift-left: TRUE ("Ready for Input") -> [w458]
    stop <- _ stop-if-true
    n218 = xnode ("FIFO Method Node")("Ready for Output"=w458) -> ("Element"=w460:u64, "Output Valid"=w461:bool)  [unwired: 1 in, 1 out]
    n219 = xnode ("FIFO Method Node")("Element"=w460, "Input Valid"=w461) -> ("Ready for Input"=w459:bool)  [unwired: 1 in, 1 out]
  }
  n220 = timed-loop {
    timing: w22 -> [_]
    timing-out: [_] -> w21
    shift-right: [w465] -> _
    shift-left: TRUE ("Ready for Input") -> [w464]
    stop <- _ stop-if-true
    n221 = xnode ("FIFO Method Node")("Ready for Output"=w464) -> ("Element"=w466:u64, "Output Valid"=w467:bool)  [unwired: 1 in, 1 out]
    n222 = xnode ("FIFO Method Node")("Element"=w466, "Input Valid"=w467) -> ("Ready for Input"=w465:bool)  [unwired: 1 in, 1 out]
  }
  n223 = node-c288(w9) -> ()
  n224 = node-c288(w23) -> ()
  n225 = node-c288(w21) -> ()
  n226 = node-c288(w34) -> ()
  n227 = node-c288() -> (w20:T5)  [unwired: 1 in]
  n228 = node-c288() -> (w26:T5)  [unwired: 1 in]
  n229 = timed-loop {
    timing: w20 -> [_]
    timing-out: [_] -> w19
    shift-right: [w470] -> _
    shift-left: TRUE ("Ready for Input") -> [w471]
    stop <- _ stop-if-true
    n230 = xnode ("FIFO Method Node")("Ready for Output"=w471) -> ("Element"=w472:cluster{"Older Data":u64, "Newer Data":u64}, "Output Valid"=w473:bool)  [unwired: 1 in, 1 out]
    n231 = xnode ("FIFO Method Node")("Element"=w472, "Input Valid"=w473) -> ("Ready for Input"=w470:bool)  [unwired: 1 in, 1 out]
  }
  n232 = timed-loop {
    timing: w26 -> [_]
    timing-out: [_] -> w25
    shift-right: [w476] -> _
    shift-left: TRUE ("Ready for Input") -> [w477]
    stop <- _ stop-if-true
    n233 = xnode ("FIFO Method Node")("Ready for Output"=w477) -> ("Element"=w478:cluster{"Older Data":u64, "Newer Data":u64}, "Output Valid"=w479:bool)  [unwired: 1 in, 1 out]
    n234 = xnode ("FIFO Method Node")("Element"=w478, "Input Valid"=w479) -> ("Ready for Input"=w476:bool)  [unwired: 1 in, 1 out]
  }
  n235 = node-c288() -> (w8:T5)  [unwired: 1 in]
  n236 = node-c288(w31) -> ()
  n237 = timed-loop {
    timing: w8 -> [_]
    timing-out: [_] -> w7
    shift-right: [w489] -> _
    shift-left: NeighbouringAvgStates."Read_noDS" ("f") -> [w488]
    shift-right: [w487] -> _
    shift-left: _ -> [w486]
    shift-right: [w483] -> _
    shift-left: TRUE ("Ready for Input") -> [w485]
    stop <- _ stop-if-true
    n238 = case shown="\"Read_noDS\", Default" w488 {
      tunnel: [w497 NeighbouringAvgStates."Write2_noDS" ("f") NeighbouringAvgStates."Read_noDS" ("f")] -> w489
      tunnel: [w493 w500 w504] -> w487
      tunnel: w486 -> [_ w500 w504]
      tunnel: [u64 0 ("Newer Data") w499 w503] -> w484
      tunnel: [FALSE ("Input Valid") w498 w502] -> w482
      tunnel: w485 -> [w490 w498 w502]
      frame "Read_noDS", Default {
        n239 = xnode ("FIFO Method Node")("Ready for Output"=w490) -> ("Element"=w493:cluster{"Older Data":u64, "Newer Data":u64}, "Output Valid"=w496:bool)  [unwired: 1 in, 1 out]
        n240 = Select(t=NeighbouringAvgStates."Write1_noDS", s=w496, f=NeighbouringAvgStates."Read_noDS") -> (s? t:f=w497:T4)
      }
      frame "Write1_noDS" {
        n241 = Unbundle By Name(w500) -> ("Older Data"=w499:u64)
      }
      frame "Write2_noDS" {
        n242 = Unbundle By Name(w504) -> ("Newer Data"=w503:u64)
      }
    }
    n243 = xnode ("FIFO Write Using Handshaking")("Element"=w484, "Input Valid"=w482) -> ("Ready for Input"=w483:bool)  [unwired: 1 in, 1 out]
  }
  n244 = node-c288(w17) -> ()
  n245 = node-c288(w19) -> ()
  n246 = node-c288(w25) -> ()
  n247 = node-c288(w7) -> ()
